vi "sat_op_fxp_16_5.vi"(8 "N_sat":u8=3, 11 "uk_in":fxp<+/-,16,5>) -> (3 "Hinv(uk)":fxp<+/-,32,10>)   [LabVIEW 2017]
uses:
  <vilib>/Platform/TimedLoop/XDataNode/timing_clust.ctl
  <vilib>/Platform/TimedLoop/XDataNode/nitl_modes.ctl
  <vilib>/Platform/TimedLoop/XDataNode/wakeup.ctl
  <vilib>/rvi/IPIntegrationNode/IPINode_Typedef/niFpgaIPINodeSupportedFamilies.ctl
  <vilib>/rvi/Emulation/niFpgaSctlEmulationGetInTimedLoop.vi
  <vilib>/rvi/Emulation/niFpgaEmulationReportErrorSimple.vi
  <vilib>/rvi/Emulation/niFpgaGetClockAttributes.vi
  <vilib>/rvi/Emulation/niFpgaCriticalErrorInLSC.vi
  <vilib>/rvi/IPIntegrationNode/IPINode_Utilities/niFpgaIPINodeSimCore.vi
  <vilib>/rvi/Memory/Memory_Emulation/nirvimemoryFastEmulation.vi
  <vilib>/rvi/Memory/Memory_Emulation/nirvimemoryEmulation.vi
  <vilib>/rvi/Emulation/niFpgaEmulationIsFPGAContextNoSignature.vi
  <vilib>/rvi/DataTransferAndStorage/Container/Common/niFpgaContainerGetUniqueNameForEmu.vi
  <vilib>/rvi/Emulation/niFpgaProcessEmulError.vi
  <vilib>/rvi/errors/nirviReportUnexpectedCaseInternalError (U32).vi
  <vilib>/Platform/TimedLoop/XDataNode/XDataNode.xnode
  <vilib>/rvi/XilinxIP/XIPIN_XNode/niFpgaXIPIN.xnode
  hysteresis_fxp_16_5/Multiply Accumulator/Multiply_Accumulator_635C28D3DC43420AADC518895231A915.dll
  <vilib>/rvi/IPIntegrationNode/IPINode_Xnode/niFpgaIPINode.xnode
  <vilib>/rvi/DataTransferAndStorage/Container/XNode/niFpgaContainer.xnode
  <vilib>/rvi/FXPMathLib/FxpSub/XNode/nifxpmath_Sub.xnode
  <vilib>/Platform/TimedLoop/XDataNode/XDNodeRunTimeDep.lvlib
  <vilib>/rvi/FXPMathLib/sim/FxpSim.dll
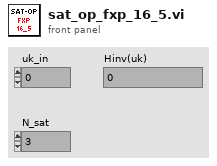
[diagram p1: front panel]
types:
  T1 = typedef "niFpgaIPINodeSupportedFamilies.ctl" = cluster{"unlimited?":bool, "supported targets":string[]}
  T2 = typedef "XDNodeRunTimeDep.lvlib/timing_clust.ctl" = cluster{"Expected End [f-1]":u64, "Actual End [f-1]":u64, "Finished Late? [f-1]":bool, "Expected End [i-1]":u64, "Actual End [i-1]":u64, "Finished Late? [i-1]":bool, "Expected Start [i]":u64, "Actual Start [i]":u64, "Expected Start [f]":u64, "Actual Start [f]":u64, "Source Name":string, "Structure Name":string, "Period":i64, "Deadline":i64, "Offset":i64, "Start":i64, "Priority":i32, "Timeout":i32, "Mode":T3, "Wakeup Reason":T4, "Error":errorcluster, "Source Type":string, "Secondary Source Type":string, "Global End Time":u64, "Global Start Time":u64, "Frame Duration":u64, "Iteration Duration":u64, "Assigned CPU":i32, "I/O Scan Engine Mode":u32}
  T3 = typedef "XDNodeRunTimeDep.lvlib/nitl_modes.ctl" = enum32{"No Change", "Process missed periods, maintain original phase", "Discard missed periods, maintain original phase", "Process missed periods, ignore original phase", "Discard missed periods, ignore original phase"}
  T4 = typedef "XDNodeRunTimeDep.lvlib/wakeup.ctl" = enum32{"Normal", "Aborted", "Asynchronous wakeup", "Timing source error", "Timed loop error", "Timeout"}
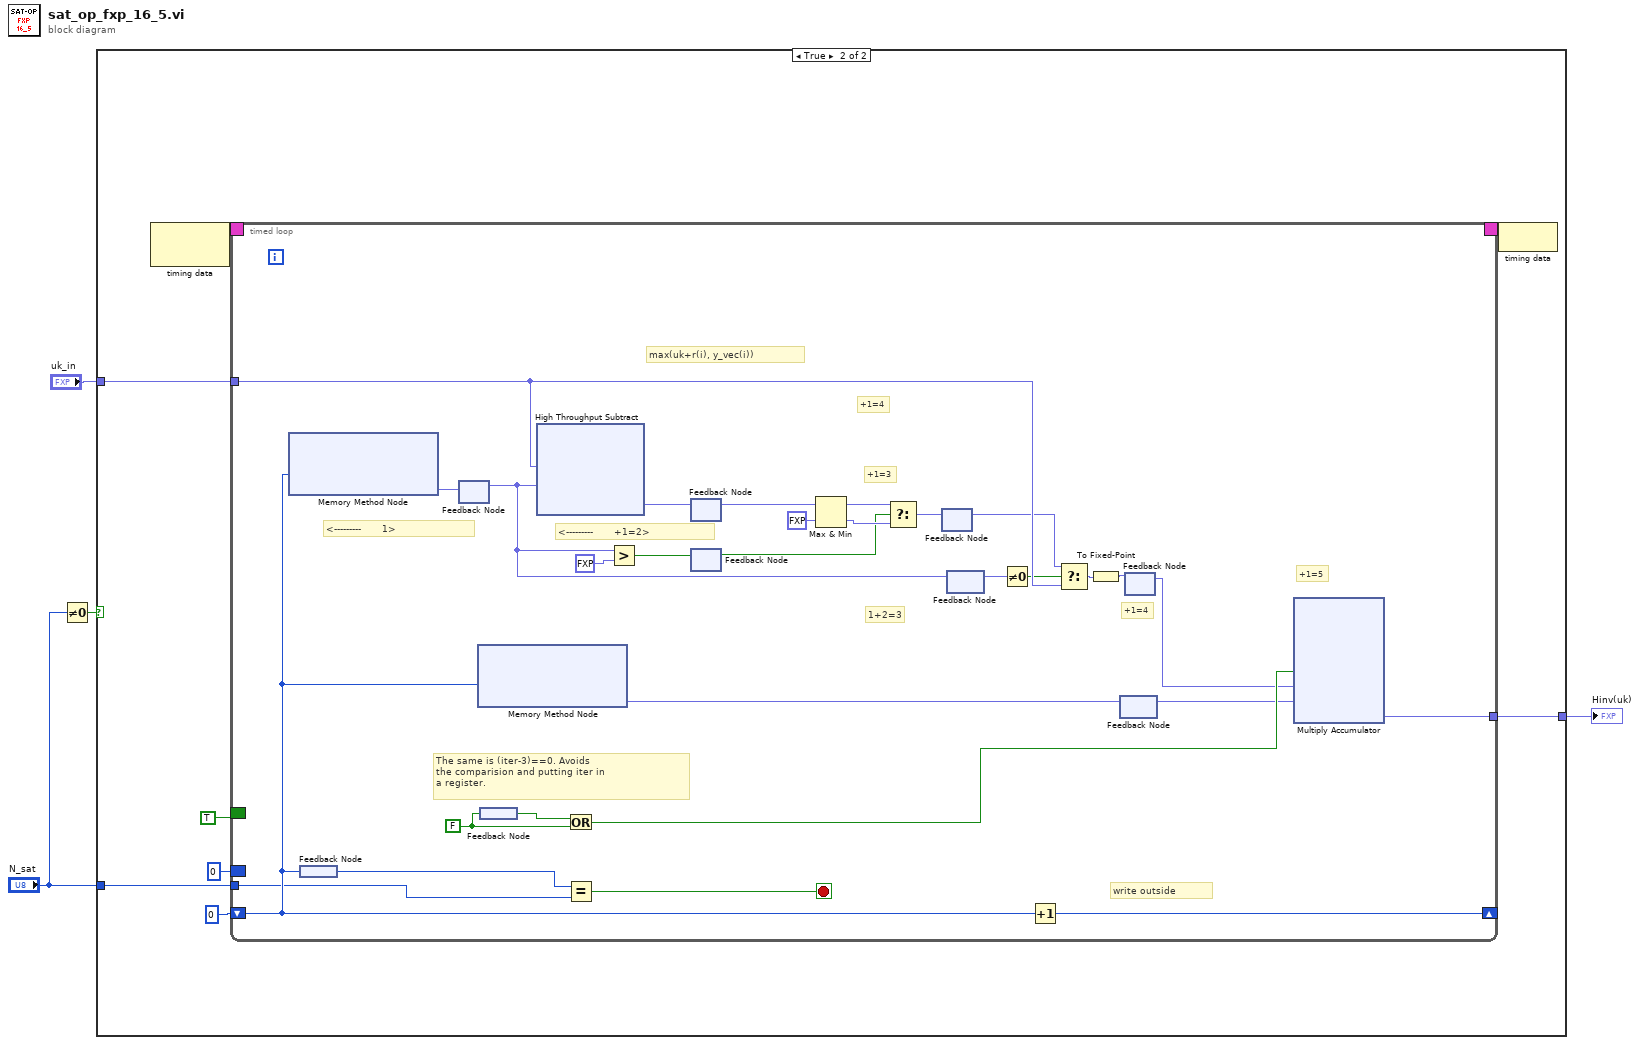
[diagram p0: block diagram]
diagram:
  n1 = Not Equal To 0?(x="N_sat") -> (x != 0?=w2:bool)
  n2 = case shown="True" w2 {
    tunnel: [w5 w9] -> w4
    tunnel: "uk_in" -> [w5 w7]
    tunnel: "N_sat" -> [_ w6]
    frame False {
    }
    frame True {
      n3 = node-c288() -> (w13:T2)  [unwired: 1 in]
      n4 = timed-loop {
        timing: w13 -> [_]
        timing-out: [_] -> w12
        tunnel: w7 -> [w33]
        border: u8 0 -> [_]
        tunnel: [w42] -> w9
        shift-right: [w40] -> _
        shift-left: u8 0 -> [w39]
        border: TRUE -> [_]
        tunnel: w6 -> [w30]
        stop <- w41 stop-if-true
        w36 = FALSE
        # "+1=4"
        # "1+2=3"
        # "The same is (iter-3)==0. Avoids \nthe comparision and putting iter in \na register."
        # "write outside"
        # "+1=5"
        # "<---------       +1=2>"
        # "+1=4"
        # "+1=3"
        # "<---------       1>"
        # "max(uk+r(i), y_vec(i))"
        n5 = xnode ("Memory Method Node")("Address"=w39) -> ("Data"=w16:fxp<+/-,16,5>)  [unwired: 1 in, 1 out]
        n6 = feedback #1() -> (w38:u8)
        n7 = feedback-in #1(w39) -> ()
        n8 = feedback #2() -> (w14:fxp<+/-,16,5>)  [unwired: 1 in]
        n9 = feedback-in #2(w16) -> ()
        n10 = xnode ("Memory Method Node")("Address"=w39) -> ("Data"=w29:fxp<+/-,16,5>)  [unwired: 1 in, 1 out]
        n11 = feedback #3() -> (w37:bool)
        n12 = feedback-in #3(w36) -> ()
        n13 = xnode "High Throughput Subtract"("x"=w33, "y"=w14) -> ("x-y"=w17:fxp<+/-,17,6>)
        n14 = Or(x=w37, y=w36) -> (x .or. y?=w31:bool)
        n15 = Equal?(x=w38, y=w30) -> (x = y?=w41:bool)
        n16 = Greater?(x=w14, y=fxp<+/-,16,5> 0.0) -> (0:w24:bool)
        n17 = feedback #4() -> (w18:fxp<+/-,17,6>)  [unwired: 1 in]
        n18 = feedback-in #4(w17) -> ()
        n19 = feedback #5() -> (w23:bool)  [unwired: 1 in]
        n20 = feedback-in #5(w24) -> ()
        n21 = Max & Min(x=w18, y=fxp<+/-,17,6> 0.0) -> (max(x,y)=w26:fxp<+/-,17,6>, min(x,y)=w25:fxp<+/-,17,6>)
        n22 = Select(t=w26, s=w23, f=w25) -> (s? t:f=w20:fxp<+/-,17,6>)
        n23 = feedback #6() -> (w19:fxp<+/-,17,6>)  [unwired: 1 in]
        n24 = feedback-in #6(w20) -> ()
        n25 = feedback #7() -> (w15:fxp<+/-,16,5>)  [unwired: 1 in]
        n26 = feedback-in #7(w14) -> ()
        n27 = Not Equal To 0?(x=w15) -> (x != 0?=w28:bool)
        n28 = Increment(x=w39) -> (x+1=w40:u8)
        n29 = Select(t=w19, s=w28, f=w33) -> (s? t:f=w32:fxp<+/-,16,5>)
        n30 = To Fixed-Point(number=w32) -> (fixed-point=w22:fxp<+/-,16,5>)  [unwired: 1 in]
        n31 = feedback #8() -> (w27:fxp<+/-,16,5>)  [unwired: 1 in]
        n32 = feedback-in #8(w29) -> ()
        n33 = feedback #9() -> (w21:fxp<+/-,16,5>)  [unwired: 1 in]
        n34 = feedback-in #9(w22) -> ()
        n35 = xnode ("Multiply Accumulator")("sclr"=w31, "a"=w21, "b"=w27) -> ("s"=w42:fxp<+/-,32,10>)  [unwired: 2 in]
      }
      n36 = node-c288(w12) -> ()
    }
  }
  "Hinv(uk)" <- w4
